vi "Configure Trigger (Normal).vi"(0 "VISA resource name":refnum<visa-resource-name>, 1 "Enable Trigger Delay (F: Disable)":bool, 5 "Trigger Source (0: Free Run)":i32(ring) items=["Free Run", "Video", "Line", "External1", "External2", "RF Burst"], 7 "Trigger Level (-20 dBm)":dbl=-20.0, 9 "Trigger Slope (0: Positive)":i32(ring) items=["Positive", "Negative"], 11 "error in (no error)":errorcluster, 12 "Trigger Delay (1E-6 s)":dbl=1e-06) -> (4 "VISA resource name out":refnum<visa-resource-name>, 15 "error out":errorcluster)   [LabVIEW 2018, in "Agilent MXA Series.lvlib"]
doc: "Configures the normal trigger settings."
uses:
  Agilent MXA Series.lvlib
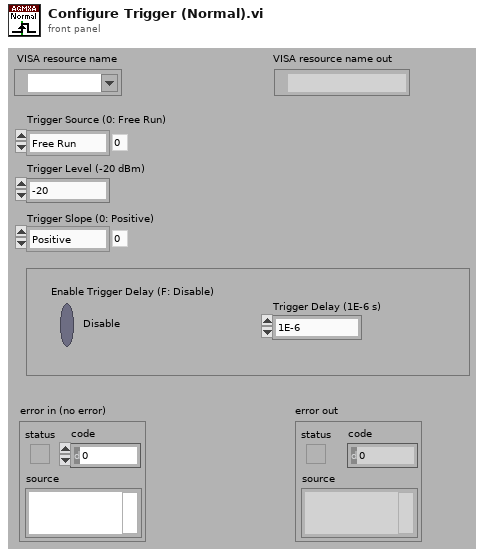
[diagram p1: front panel]
types:
  T1 = typedef "Agilent MXA Series.lvlib/Extended User Data.ctl" = cluster{"Measurement Type":i32, "Agilent MXA/EXA Model":i32}
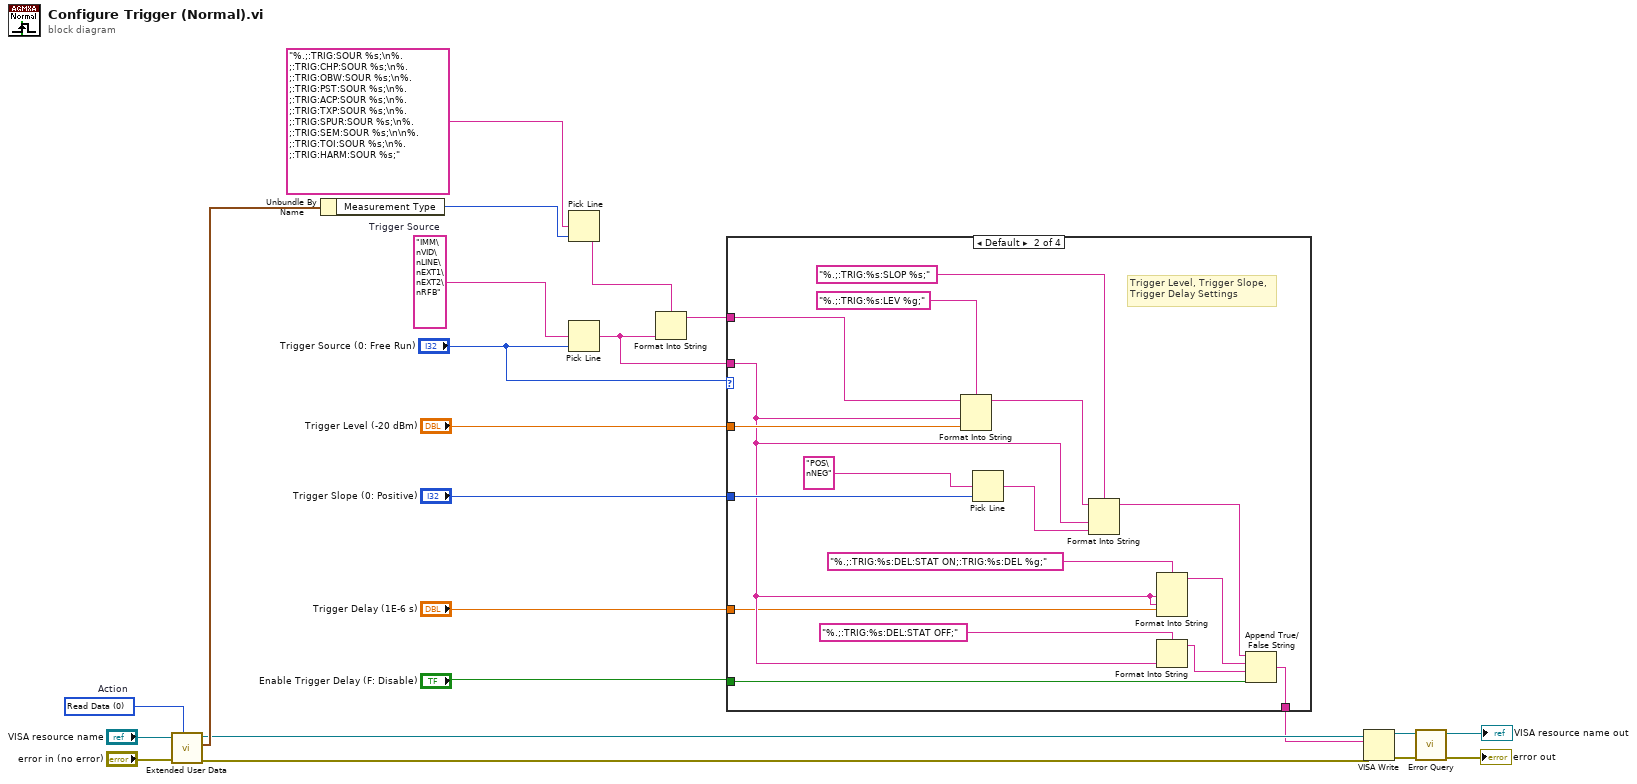
[diagram p0: block diagram]
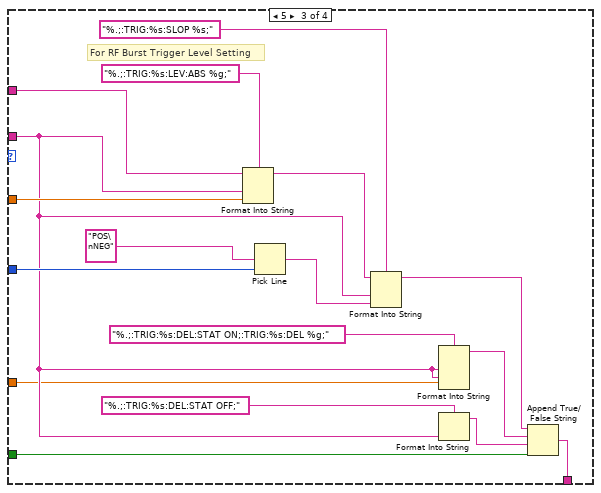
[diagram p3: hidden frame]
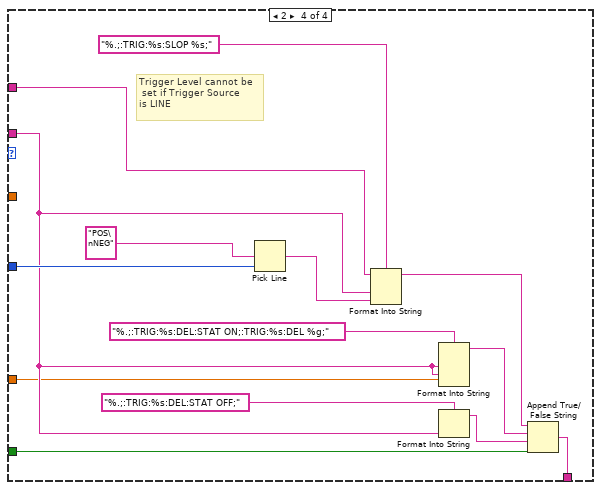
[diagram p4: hidden frame]
diagram:
  w18 = "IMM\nVID\nLINE\nEXT1\nEXT2\nRFB"  # Trigger Source
  w20 = 0 items=["Read Data", "Write Data", "Clear Data", "Clear ALL Data"]  # Action
  n1 = call "Extended User Data.vi"("Action (1:Write Data)"=w20, "Error In (no error)"="error in (no error)", "VISA resource name in"="VISA resource name") -> ("Error Out"=w17:errorcluster, "User Data Out"=w19:T1, "VISA resource name out"=w9:refnum<visa-resource-name>)  [unwired: 6 in]
  n2 = Unbundle By Name(w19) -> ("Measurement Type"=w11:i32)
  n3 = Pick Line(multi-line string="%.;:TRIG:SOUR %s;\n%.;:TRIG:CHP:SOUR %s;\n%.;:TRIG:OBW:SOUR %s;\n%.;:TRIG:PST:SOUR %s;\n%.;:TRIG:ACP:SOUR %s;\n%.;:TRIG:TXP:SOUR %s;\n%.;:TRIG:SPUR:SOUR %s;\n%.;:TRIG:SEM:SOUR %s;\n\n%.;:TRIG:TOI:SOUR %s;\n%.;:TRIG:HARM:SOUR %s;", line index=w11) -> (output string=w10:string)  [unwired: 1 in]
  n4 = Pick Line(multi-line string=w18, line index="Trigger Source (0: Free Run)") -> (output string=w2:string)  [unwired: 1 in]
  n5 = Format Into String(format string=w10, w2) -> (resulting string=w3:string)  [unwired: 2 in, 1 out]
  n6 = case shown="Default" "Trigger Source (0: Free Run)" {
    tunnel: "Enable Trigger Delay (F: Disable)" -> [_ w28 w45 w63]
    tunnel: "Trigger Delay (1E-6 s)" -> [_ w29 w46 w64]
    tunnel: "Trigger Slope (0: Positive)" -> [_ w36 w53 w70]
    tunnel: "Trigger Level (-20 dBm)" -> [_ w38 w55 _]
    tunnel: w3 -> [w23 w39 w56 w58]
    tunnel: w2 -> [_ w30 w47 w65]
    tunnel: [w23 w24 w41 w59] -> w1
    frame 0 {
      # "If trigger source is free run, no trigger property needs to be set"
    }
    frame Default {
      # "Trigger Level, Trigger Slope,\nTrigger Delay Settings"
      n7 = Format Into String(format string="%.;:TRIG:%s:LEV %g;", initial string=w39, w30, w38) -> (resulting string=w33:string)  [unwired: 1 in, 1 out]
      n8 = Pick Line(multi-line string="POS\nNEG", line index=w36) -> (output string=w35:string)  [unwired: 1 in]
      n9 = Format Into String(format string="%.;:TRIG:%s:SLOP %s;", initial string=w33, w30, w35) -> (resulting string=w25:string)  [unwired: 1 in, 1 out]
      n10 = Format Into String(format string="%.;:TRIG:%s:DEL:STAT ON;:TRIG:%s:DEL %g;", w30, w30, w29) -> (resulting string=w27:string)  [unwired: 2 in, 1 out]
      n11 = Format Into String(format string="%.;:TRIG:%s:DEL:STAT OFF;", w30) -> (resulting string=w26:string)  [unwired: 2 in, 1 out]
      n12 = Append True/False String(1:w28, 2:w26, 3:w27, 4:w25) -> (0:w24:string)
    }
    frame 5 {
      # "For RF Burst Trigger Level Setting"
      n13 = Format Into String(format string="%.;:TRIG:%s:LEV:ABS %g;", initial string=w56, w47, w55) -> (resulting string=w50:string)  [unwired: 1 in, 1 out]
      n14 = Pick Line(multi-line string="POS\nNEG", line index=w53) -> (output string=w52:string)  [unwired: 1 in]
      n15 = Format Into String(format string="%.;:TRIG:%s:SLOP %s;", initial string=w50, w47, w52) -> (resulting string=w42:string)  [unwired: 1 in, 1 out]
      n16 = Format Into String(format string="%.;:TRIG:%s:DEL:STAT ON;:TRIG:%s:DEL %g;", w47, w47, w46) -> (resulting string=w44:string)  [unwired: 2 in, 1 out]
      n17 = Format Into String(format string="%.;:TRIG:%s:DEL:STAT OFF;", w47) -> (resulting string=w43:string)  [unwired: 2 in, 1 out]
      n18 = Append True/False String(1:w45, 2:w43, 3:w44, 4:w42) -> (0:w41:string)
    }
    frame 2 {
      # "Trigger Level cannot be\n set if Trigger Source \nis LINE"
      n19 = Pick Line(multi-line string="POS\nNEG", line index=w70) -> (output string=w69:string)  [unwired: 1 in]
      n20 = Format Into String(format string="%.;:TRIG:%s:SLOP %s;", initial string=w58, w65, w69) -> (resulting string=w60:string)  [unwired: 1 in, 1 out]
      n21 = Format Into String(format string="%.;:TRIG:%s:DEL:STAT ON;:TRIG:%s:DEL %g;", w65, w65, w64) -> (resulting string=w62:string)  [unwired: 2 in, 1 out]
      n22 = Format Into String(format string="%.;:TRIG:%s:DEL:STAT OFF;", w65) -> (resulting string=w61:string)  [unwired: 2 in, 1 out]
      n23 = Append True/False String(1:w63, 2:w61, 3:w62, 4:w60) -> (0:w59:string)
    }
  }
  n24 = VISA Write(VISA resource name=w9, write buffer=w1, error in (no error)=w17) -> (VISA resource name out=w16:refnum<visa-resource-name>, error out=w15:errorcluster)  [unwired: 1 out]
  n25 = call "Error Query.vi"("error in (no error)"=w15, "VISA resource name"=w16) -> ("error out"=→"error out":errorcluster, "VISA resource name out"=→"VISA resource name out":refnum<visa-resource-name>)  [unwired: 6 in, 2 out]
